vi "PlotGraph.vi"(5 "Waveform Graph":refnum<vi>, 7 "Graph":refnum<vi>, 9 "Channel array":refnum<vi>[](array[refnum]), 10 "Amplitude array":refnum<vi>[](array[refnum]), 11 "Polarity array":refnum<vi>[](array[refnum])) -> (2 "Cursor Position":T1 min=-999.0 max=999.0 format="%+.12f")   [LabVIEW 2009]
uses:
  DelayControl2.ctl
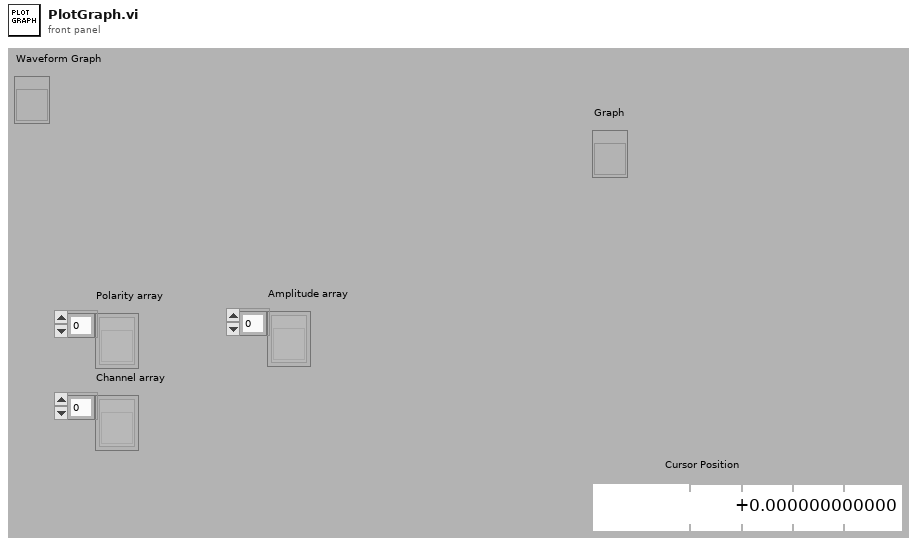
[diagram p1: front panel]
types:
  T1 = typedef "DelayControl2.ctl" = dbl
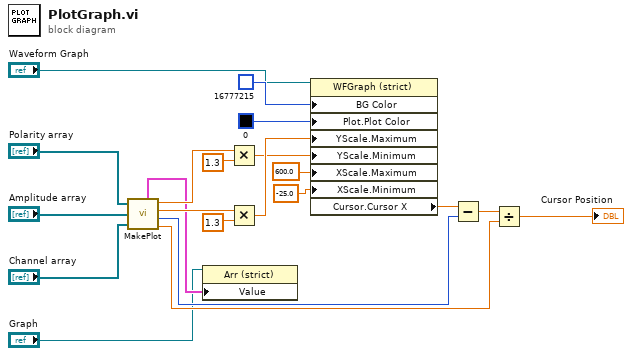
[diagram p0: block diagram]
diagram:
  n1 = call "MakePlot.vi"("Polarity array"="Polarity array", "Amplitude array"="Amplitude array", "Channel array"="Channel array") -> ("Numeric 2"=w14:dbl, "Numeric 3"=w18:dbl, "samples"=w9:i32, "Numeric"=w7:T1, "Array"=w3:cluster{"Pulse Pattern":dbl[]}[])
  n2 = property class="Arr (strict)"(reference="Graph", "Value"=w3) -> ()  [unwired: 1 in, 2 out]
  n3 = Multiply(x=w14, y=1.3) -> (x*y=w13:dbl)
  n4 = Multiply(x=w18, y=1.3) -> (x*y=w15:dbl)
  n5 = property class="WFGraph (strict)"(reference="Waveform Graph", "BG Color"=u32 16777215 ("Color"), "Plot.Plot Color"=u32 0 ("Color"), "YScale.Maximum"=w15, "YScale.Minimum"=w13, "XScale.Maximum"=600.0 ("X Scale.Range:Maximum"), "XScale.Minimum"=-25.0 ("X Scale.Range:Minimum")) -> ("Cursor.Cursor X"=w10:dbl)  [unwired: 1 in, 2 out]
  n6 = Subtract(x=w10, y=w9) -> (x-y=w8:dbl)
  n7 = Divide(x=w8, y=w7) -> (x/y=→"Cursor Position":T1)
